vi "CopyResultsFile.vi"(8 "error in (no error)":errorcluster, 9 "Wheelname":string, 10 "Server Path":path, 11 "source path":path) -> (0 "error out":errorcluster)   [LabVIEW 2013]
doc: "Use this template to build a VI to use as a subVI."
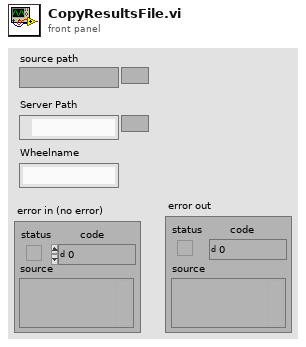
[diagram p1: front panel]
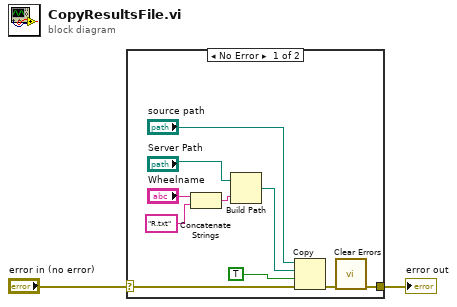
[diagram p0: block diagram]
diagram:
  n1 = case shown="No Error" "error in (no error)" {
    selector: "error in (no error)" -> [w11 w13]
    tunnel: [w7 w13] -> w1
    frame No Error {
      n2 = Concatenate Strings("Wheelname", "R.txt") -> (w3:string)
      n3 = Build Path(base path="Server Path", name or relative path=w3) -> (appended path=w9:path)
      n4 = Copy(8:w11, 9:TRUE ("overwrite (F)"), 10:w9, 11:"source path") -> (0:w8:errorcluster)  [unwired: 1 in, 2 out]
      n5 = call <vilib>:"Clear Errors.vi"("error in (no error)"=w8) -> ("error out"=w7:errorcluster)  [unwired: 6 in]
    }
    frame Error {
    }
  }
  "error out" <- w1
